vi "string send.vi"() -> ()   [LabVIEW 2011]
uses:
  <vilib>/LabVIEW Interface for Arduino/LabVIEW Interface for Arduino.lvlib
  <vilib>/LabVIEW Interface for Arduino/Type Defs/Connection Type.ctl
  <vilib>/LabVIEW Interface for Arduino/Type Defs/Board Type.ctl
panel:
  in  "Tab Control":enum32{"Settings", "Page 2"}(tab)
  in  "VISA resource name":refnum<visa-resource-name>
  in  "Stop Button":bool
  in  "Baud Rate":u32
  in  "Connection Type":T1
  in  "Board Type":T2
  out "Error Out":errorcluster
  in  "Base (String)":T3(ring)
  in  "String":string
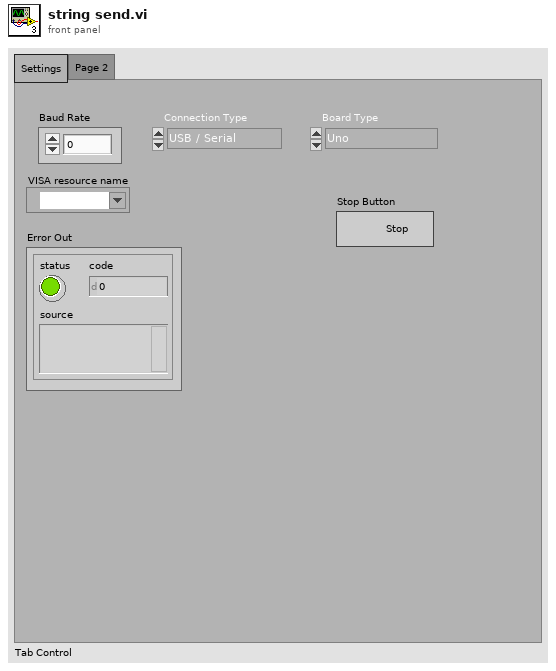
[diagram p1: front panel]
types:
  T1 = typedef "LabVIEW Interface for Arduino.lvlib/Connection Type.ctl" = enum8{"USB / Serial", "XBEE", "BlueSmirf (Bluetooth)"}
  T2 = typedef "LabVIEW Interface for Arduino.lvlib/Board Type.ctl" = enum16{"Uno", "Dimuelanove w/Atmega 328", "Mega 2560"}
  T3 = enum8{"String", "Binary", "Decimal", "Octal", "Hexadecimal"}
  T4 = typedef "LabVIEW Interface for Arduino.lvlib/Arduino Resource.ctl" = cluster{"VISA resource":refnum<visa-resource-name>, "Board Type":T2, "Connection Type":enum8{"USB / Serial"}, "Bytes Per Packet (15)":u8}
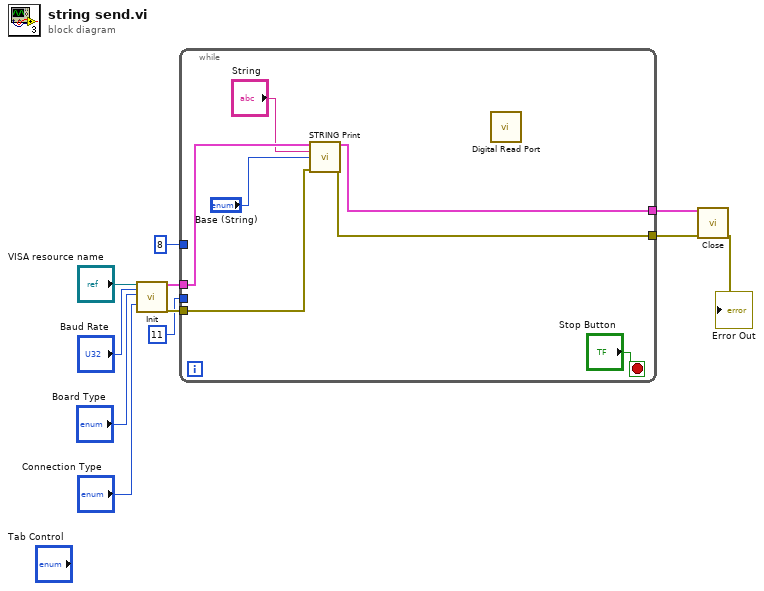
[diagram p0: block diagram]
diagram:
  n1 = call <vilib>:"Init.vi"("VISA resource"="VISA resource name", "Baud Rate (115200)"="Baud Rate", "Board Type (Uno)"="Board Type", "Connection Type (USB/Serial)"="Connection Type") -> ("Arduino Resource"=w8:T4, "error out"=w7:errorcluster)  [unwired: 14 in]
  n2 = while {
    tunnel: w8 -> [w17]
    tunnel: w7 -> [w16]
    tunnel: 11 -> [_]
    tunnel: 8 -> [_]
    tunnel: [w13] -> w2
    tunnel: [w12] -> w1
    stop <- "Stop Button" stop-if-true
    n3 = call <vilib>:"STRING Print.vi"("Arduino Resource"=w17, "Data"="String", "Base (String)"="Base (String)", "error out"=w16) -> ("Arduino Resource"=w13:T4, "error out"=w12:errorcluster)  [unwired: 10 in]
    n4 = call <vilib>:"Digital Read Port.vi"() -> ()  [unwired: 13 in, 3 out]
  }
  n5 = call <vilib>:"Close.vi"("Arduino Resource"=w2, "error in"=w1) -> ("error out"=→"Error Out":errorcluster)  [unwired: 13 in]
